vi "DevNum_StartAndSpan.vi"(9 "Device number":i32, 10 "DevNums":i32[](array[numeric])=[0, 0, 0, 0, 0, 0, 0, 0, 0, 0, 0, 0, 0, 0, 0, 0, 0, 0, 0, 0, 0, 0, 0, 0, 0, 0, 0, 0, 0, 0, 1, 1, 1, 1, 1, 1, 1, 1, 1, 1, 1, 1, 1, 1, 1, 1, 1, 1, 1, 1, 2, 2, 2, 2, 2, 2, 2, 2, 2, 2, 2, 2, 2, 2, 2, 2, 2, 2, 2, 2, 3, 3, 3, 3, 3, 3, 3, 3, 3, 3, 3, 3, 3, 3, 3, 3, 3, 3, 3, 3, 4, 4, 4, 4, 4, 4, 4, 4, 5, 5, 5, 5, 5, 5, 5, 5, 5, 5, 5, 5, 6, 6, 6, 6, 6, 6, 6, 6, 6, 6, 6, 6, 7, 7, 7, 7, 7, 7, 7, 7, 7, 7, 7, 7]) -> (1 "start col index":i32, 2 "num cols":i32)   [LabVIEW 2013]
doc: "Get start and span of a particular \"device number\" in DevNums array. If the device number is not found, start-> -1 and span -> 0. Note: validity of DevNums (consecutive, only increasing) is not checked."
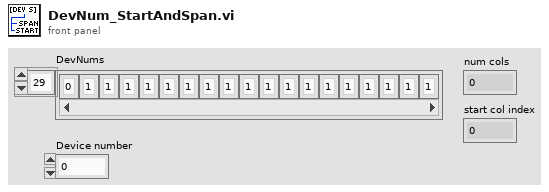
[diagram p1: front panel]
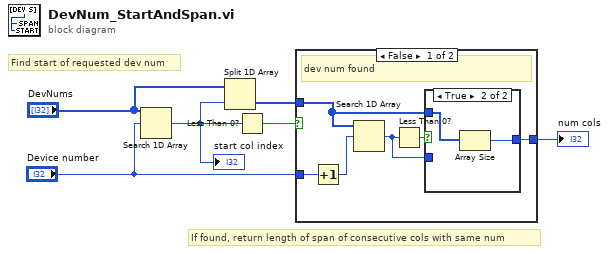
[diagram p0: block diagram]
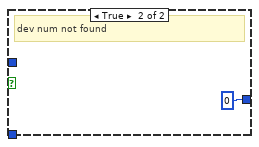
[diagram p3: hidden frame]
diagram:
  # "If found, return length of span of consecutive cols with same num"
  # "Find start of requested dev num"
  n1 = Search 1D Array(1D array="DevNums", element="Device number") -> (index of element=w2:i32)  [unwired: 1 in]
  "start col index" <- w2
  n2 = Split 1D Array(array="DevNums", index=w2) -> (second subarray=w4:i32[])  [unwired: 1 out]
  n3 = Less Than 0?(x=w2) -> (x < 0?=w1:bool)
  n4 = case shown="False" w1 {
    tunnel: "Device number" -> [w12 _]
    tunnel: w4 -> [w8 _]
    tunnel: [w7 0] -> w3
    frame False {
      # "dev num found"
      n5 = Increment(x=w12) -> (x+1=w11:i32)
      n6 = Search 1D Array(1D array=w8, element=w11) -> (index of element=w9:i32)  [unwired: 1 in]
      n7 = Less Than 0?(x=w9) -> (x < 0?=w10:bool)
      n8 = case shown="True" w10 {
        tunnel: w9 -> [w13 _]
        tunnel: w8 -> [_ w15]
        tunnel: [w13 w14] -> w7
        frame False {
        }
        frame True {
          n9 = Array Size(array=w15) -> (size(s)=w14:i32)
        }
      }
    }
    frame True {
      # "dev num not found"
    }
  }
  "num cols" <- w3
